vi "Channels to Block Conversions.vi"(11 "Transfer Configuration":T1 {"channels"."string offset" format="%d bytes"}) -> (3 "Transfer conversion descriptors":T6[](array[typedef]) {"string offset" format="%d bytes"; "engine offset" format="%d bytes"})   [LabVIEW 2017, in "String Type Converter.lvlib" / "String Type Converter.lvclass"]
uses:
  String Type Converter.lvclass
  Conversion Block.ctl
  Builds/Data Sharing Framework/Current/Core/DSF Core.lvlibp/Typedefs/DSF Data Type.ctl
  Builds/Data Sharing Framework/Current/Core/DSF Core.lvlibp/Typedefs/DSF Engine Transfer Configuration.ctl
  Builds/Data Sharing Framework/Current/Core/DSF Core.lvlibp/Typedefs/DSF Byte Order.ctl
  Builds/Data Sharing Framework/Current/Core/DSF Core.lvlibp/Typedefs/DSF Settings Info.ctl
  Builds/Data Sharing Framework/Current/Core/DSF Core.lvlibp/Typedefs/DSF Engine Channel Configuration.ctl
  Builds/Data Sharing Framework/Current/Core/DSF Core.lvlibp
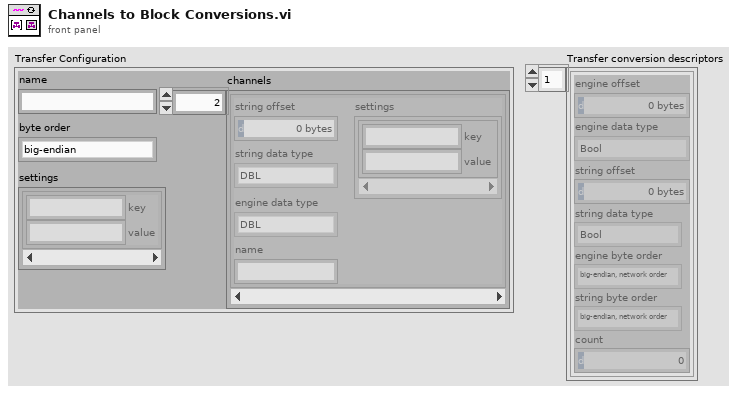
[diagram p1: front panel]
types:
  T1 = typedef "DSF Core.lvlibp/DSF Engine Transfer Configuration.ctl" = cluster{"name":string, "byte order":T2, "settings":T3, "channels":T4[]}
  T2 = typedef "DSF Core.lvlibp/DSF Byte Order.ctl" = enum8{"big-endian", "little-endian"}
  T3 = typedef "DSF Core.lvlibp/DSF Settings Info.ctl" = cluster{"key":string, "value":string}[]
  T4 = typedef "DSF Core.lvlibp/DSF Engine Channel Configuration.ctl" = cluster{"string offset":u64, "string data type":T5, "engine data type":T5, "name":string, "settings":T3}
  T5 = typedef "DSF Core.lvlibp/DSF Data Type.ctl" = enum8{"Bool", "SGL", "DBL", "I8", "I16", "I32", "I64", "U8", "U16", "U32", "U64"}
  T6 = typedef "String Type Converter.lvlib/String Type Converter.lvclass/Conversion Block.ctl" = cluster{"engine offset":u64, "engine data type":T5, "string offset":u64, "string data type":T5, "engine byte order":enum16{"big-endian, network order", "native, host order", "little-endian"}, "string byte order":enum16{"big-endian, network order", "native, host order", "little-endian"}, "count":u64}
  T7 = enum16{"big-endian, network order", "native, host order", "little-endian"}
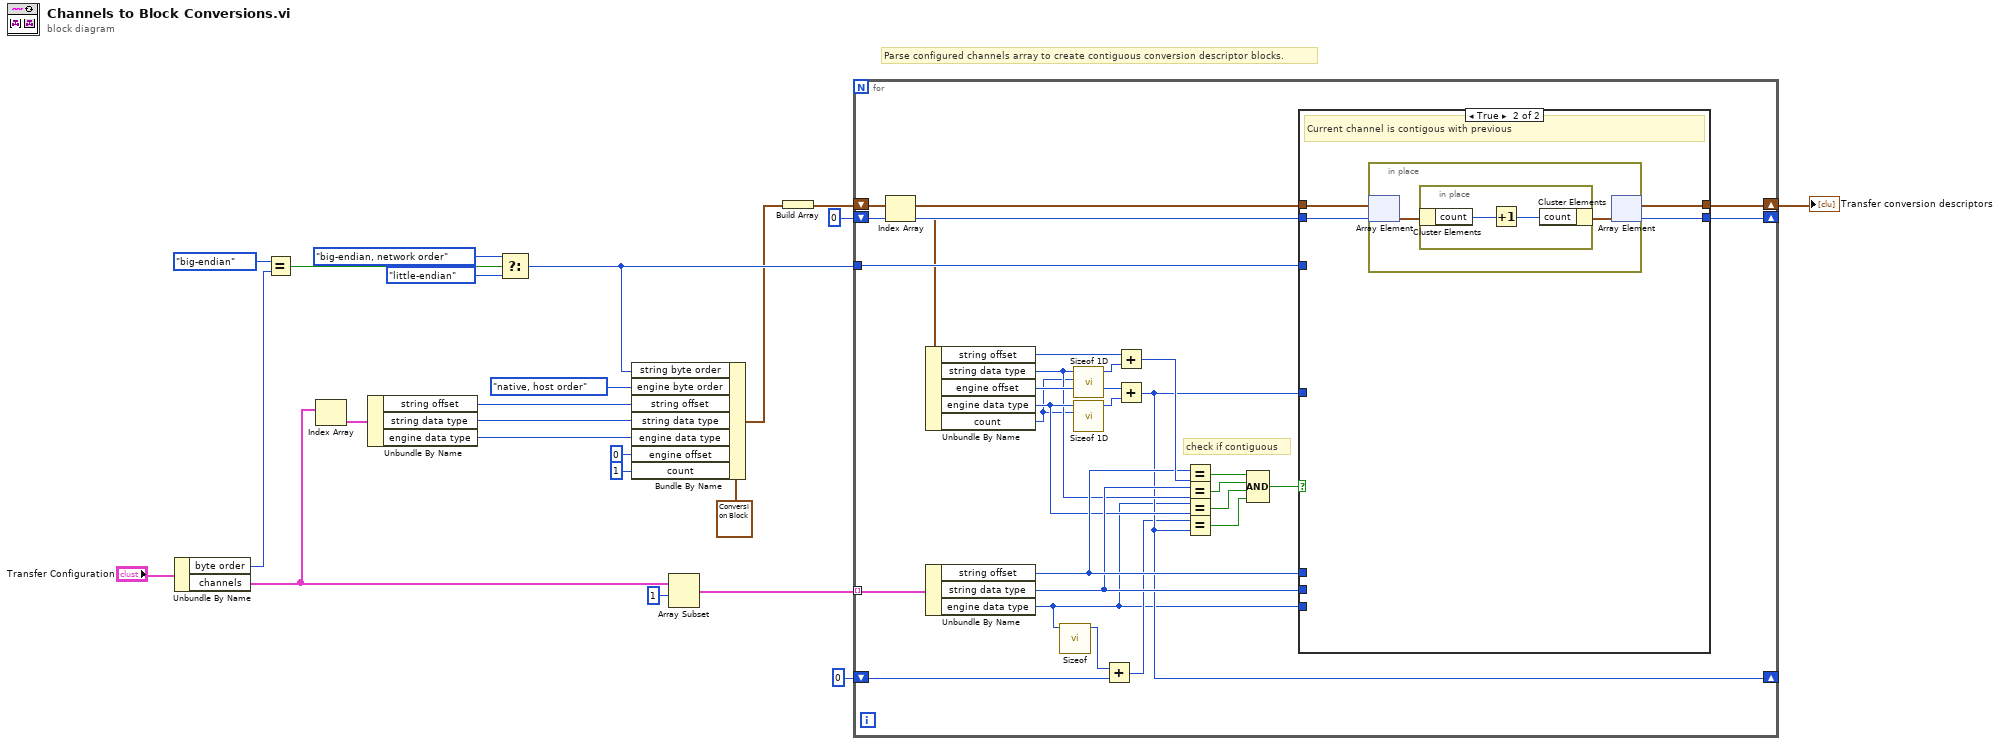
[diagram p0: block diagram]
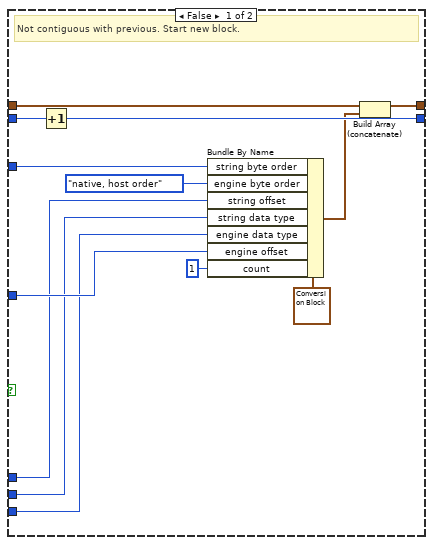
[diagram p2: hidden frame]
diagram:
  # "Parse configured channels array to create contiguous conversion descriptor blocks."
  n1 = Unbundle By Name("Transfer Configuration") -> ("byte order"=w18:T2, "channels"=w9:T4[])
  n2 = Equal?(x=DSF_Byte_Order."big-endian", y=w18) -> (x = y?=w22:bool)
  n3 = Index Array(array=w9) -> (element=w8:T4)  [unwired: 1 in]
  n4 = Unbundle By Name(w8) -> ("string offset"=w11:u64, "string data type"=w10:T5, "engine data type"=w2:T5)
  n5 = Select(t=T7."big-endian, network order" ("engine byte order"), s=w22, f=T7."little-endian" ("engine byte order")) -> (s? t:f=w15:T7)
  n6 = Bundle By Name(cluster=T6 {"engine offset"=0, "engine data type"=enum."Bool", "string offset"=0, "string data type"=enum."Bool", "engine byte order"=enum."big-endian, network order", "string byte order"=enum."big-endian, network order", "count"=0} ("conversion descriptor"), "string byte order"=w15, "engine byte order"=T7."native, host order", "string offset"=w11, "string data type"=w10, "engine data type"=w2, "engine offset"=u64 0, "count"=u64 1) -> (w4:T6)
  n7 = Array Subset(array=w9, index=1) -> (w12:T4[])  [unwired: 1 in]
  n8 = Build Array(w4) -> (w3:T6[])
  n9 = for {
    tunnel: w12 -> [w50] mode=indexing
    tunnel: w15 -> [w49]
    shift-right: [w29] -> _
    shift-left: u64 0 -> [w26]
    shift-right: [w34] -> w6
    shift-left: w3 -> [w32]
    shift-right: [w33] -> _
    shift-left: 0 -> [w31]
    # "check if contiguous"
    n10 = Index Array(array=w32, index=w31) -> (element=w30:T6)
    n11 = Unbundle By Name(w30) -> ("string offset"=w47:u64, "string data type"=w35:T5, "engine offset"=w36:u64, "engine data type"=w37:T5, "count"=w28:u64)
    n12 = Unbundle By Name(w50) -> ("string offset"=w39:u64, "string data type"=w38:T5, "engine data type"=w24:T5)
    n13 = call "Sizeof.vi"("data type"=w24) -> ("size in bytes"=w27:u64)  [unwired: 9 in, 1 out]
    n14 = call "Sizeof 1D.vi"("count"=w28, "data type"=w35) -> ("size in bytes"=w46:u64)  [unwired: 9 in]
    n15 = call "Sizeof 1D.vi"("count"=w28, "data type"=w37) -> ("size in bytes"=w48:u64)  [unwired: 9 in]
    n16 = Add(x=w27, y=w26) -> (x+y=w25:u64)
    n17 = Add(x=w47, y=w46) -> (x+y=w45:u64)
    n18 = Add(x=w36, y=w48) -> (x+y=w29:u64)
    n19 = Equal?(x=w39, y=w45) -> (x = y?=w44:bool)
    n20 = Equal?(x=w38, y=w35) -> (x = y?=w41:bool)
    n21 = Equal?(x=w24, y=w37) -> (x = y?=w42:bool)
    n22 = Equal?(x=w25, y=w29) -> (x = y?=w43:bool)
    n23 = Compound Arithmetic op=AND(w44, w41, w42, w43) -> (w40:bool)
    n24 = case shown="True" w40 {
      tunnel: w24 -> [w57 _]
      tunnel: w38 -> [w56 _]
      tunnel: w39 -> [w58 _]
      tunnel: w29 -> [w59 _]
      tunnel: w49 -> [w61 _]
      tunnel: w32 -> [w53 w67]
      tunnel: [w52 w64] -> w34
      tunnel: w31 -> [w55 w66]
      tunnel: [w54 w65] -> w33
      frame False {
        # "Not contiguous with previous. Start new block."
        n25 = Increment(x=w55) -> (x+1=w54:i32)
        n26 = Bundle By Name(cluster=T6 {"engine offset"=0, "engine data type"=enum."Bool", "string offset"=0, "string data type"=enum."Bool", "engine byte order"=enum."big-endian, network order", "string byte order"=enum."big-endian, network order", "count"=0} ("conversion descriptor"), "string byte order"=w61, "engine byte order"=T7."native, host order", "string offset"=w58, "string data type"=w56, "engine data type"=w57, "engine offset"=w59, "count"=u64 1) -> (w51:T6)
        n27 = Build Array (concatenate)(w53, w51) -> (w52:T6[])
      }
      frame True {
        # "Current channel is contigous with previous"
        n28 = in-place {
          n29 = in-place-array #1(w67, w66) -> (w68:T6)
          n30 = in-place {
            n31 = in-place-cluster #2(w68) -> ("count"=w71:u64)
            n32 = Increment(x=w71) -> (x+1=w70:u64)
            n33 = in-place-cluster #2("count"=w70) -> (w69:T6)
          }
          n34 = in-place-array #1(w69) -> (w64:T6[], w65:i32)
        }
      }
    }
  }
  "Transfer conversion descriptors" <- w6
